vi "CorrectPodControlTimestep.vi"(0 "Default timestep":dbl, 1 "Drive Motor Characteristics":T2, 2 "Pod Configuration":T3, 5 "Drive Torque":dbl, 7 "Turret Motor Characteristics":T2, 9 "Loss Torque":dbl, 11 "Drive Linear Magnitude":dbl, 12 "Turret Angle Change":dbl, 13 "Turret Torque":dbl, 14 "Turret acceleration":dbl) -> (4 "Corrected Timestep":dbl, 6 "Output States":T1)   [LabVIEW 2014]
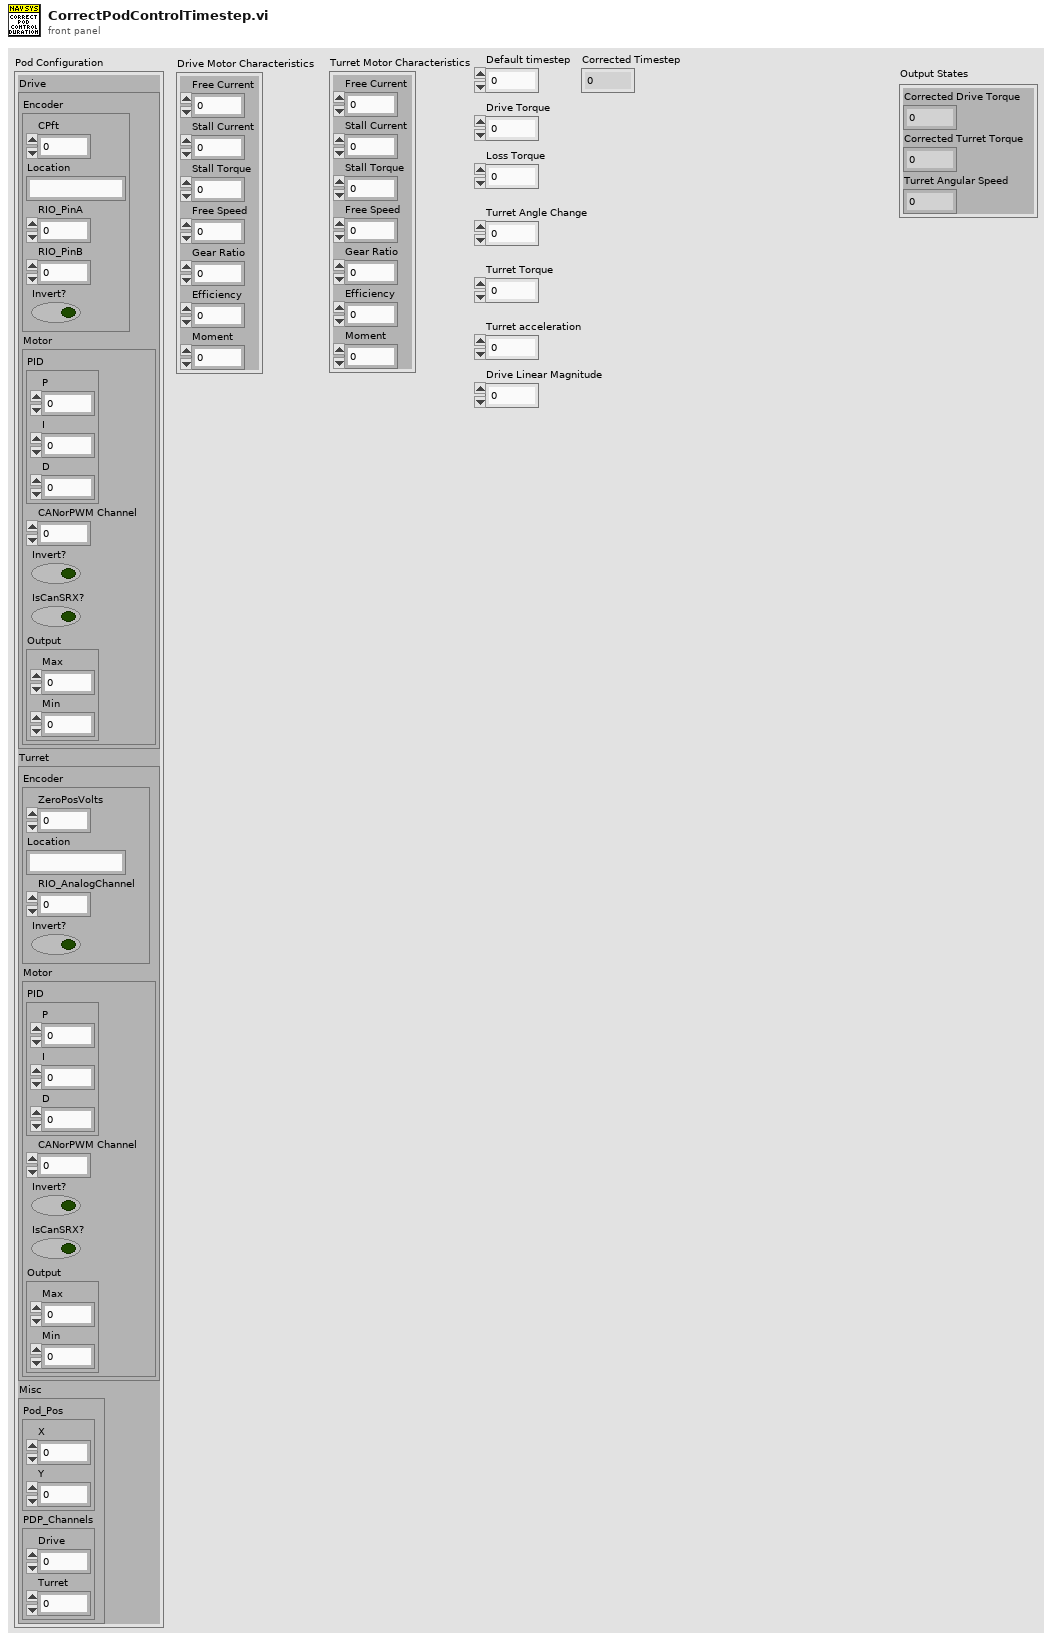
[diagram p1: front panel]
types:
  T1 = cluster{"Corrected Drive Torque":dbl, "Corrected Turret Torque":dbl, "Turret Angular Speed":dbl}
  T2 = cluster{"Free Current":dbl, "Stall Current":dbl, "Stall Torque":dbl, "Free Speed":dbl, "Gear Ratio":dbl, "Efficiency":dbl, "Moment":dbl}
  T3 = cluster{"Drive":cluster{"Encoder":cluster{"CPft":dbl, "Location":string, "RIO_PinA":i32, "RIO_PinB":i32, "Invert?":bool}, "Motor":cluster{"PID":cluster{"P":dbl, "I":dbl, "D":dbl}, "CANorPWM Channel":i32, "Invert?":bool, "IsCanSRX?":bool, "Output":cluster{"Max":dbl, "Min":dbl}}}, "Turret":cluster{"Encoder":cluster{"ZeroPosVolts":dbl, "Location":string, "RIO_AnalogChannel":i32, "Invert?":bool}, "Motor":cluster{"PID":cluster{"P":dbl, "I":dbl, "D":dbl}, "CANorPWM Channel":i32, "Invert?":bool, "IsCanSRX?":bool, "Output":cluster{"Max":dbl, "Min":dbl}}}, "Misc":cluster{"Pod_Pos":cluster{"X":dbl, "Y":dbl}, "PDP_Channels":cluster{"Drive":i32, "Turret":i32}}}
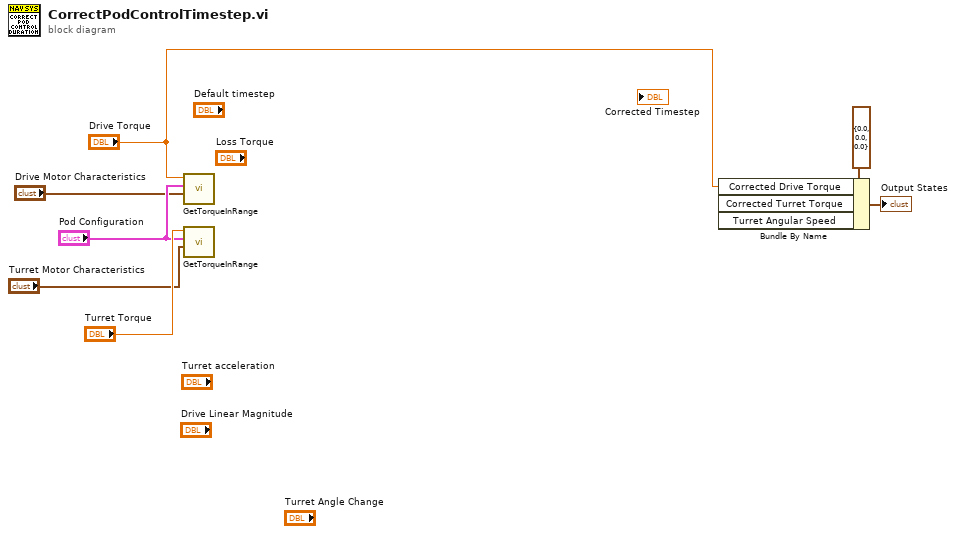
[diagram p0: block diagram]
diagram:
  n1 = call "GetTorqueInRange"("Motor Characteristics"="Drive Motor Characteristics", "Pod Configuration"="Pod Configuration", "Torque"="Drive Torque") -> ()  [unwired: 7 in, 2 out]
  n2 = call "GetTorqueInRange"("Motor Characteristics"="Turret Motor Characteristics", "Pod Configuration"="Pod Configuration", "Torque"="Turret Torque") -> ()  [unwired: 7 in, 2 out]
  n3 = Bundle By Name(cluster=T1 {"Corrected Drive Torque"=0.0, "Corrected Turret Torque"=0.0, "Turret Angular Speed"=0.0} ("Output States 2"), "Corrected Drive Torque"="Drive Torque") -> (→"Output States":T1)  [unwired: 2 in]
